vi "倒计时器.vi"() -> ()   [LabVIEW 2017]
panel:
  out "倒计时":string
  in  "停止":bool
  out "?":bool
  in  "开始倒计时":bool
  in  "定时时间选择":enum16{"20秒", "10秒", "6秒"}(ring)
  # "倒计时器"
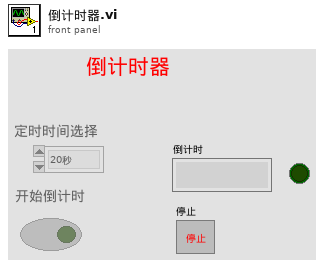
[diagram p1: front panel]
types:
  T1 = enum8{"Enabled", "Disabled", "Disabled and Grayed Out"}
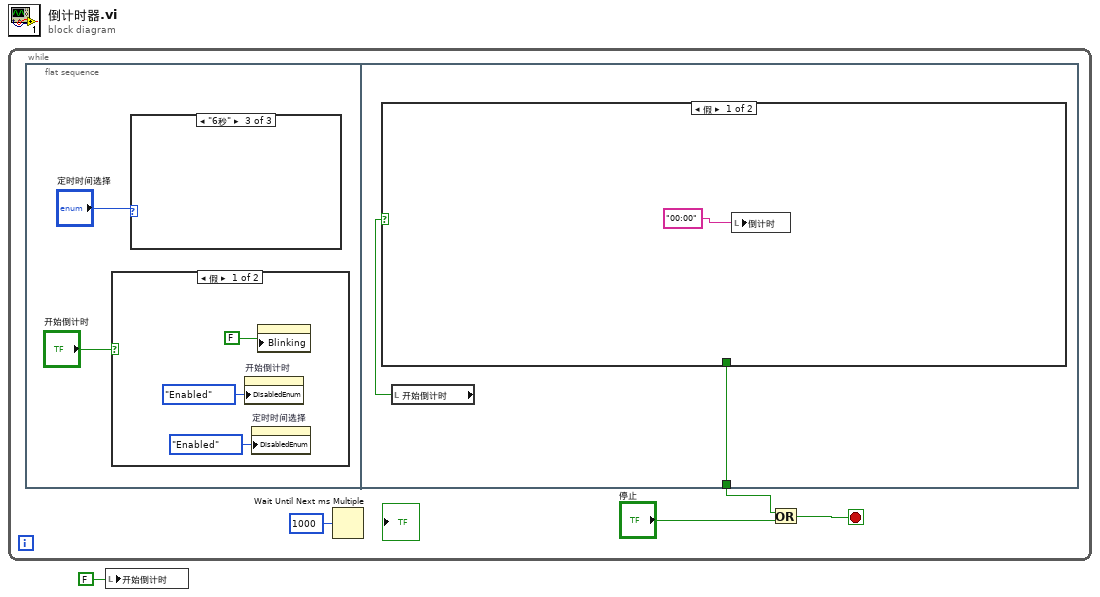
[diagram p0: block diagram]
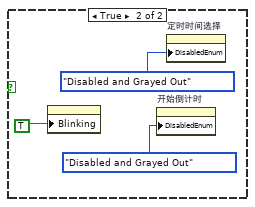
[diagram p2: hidden frame]
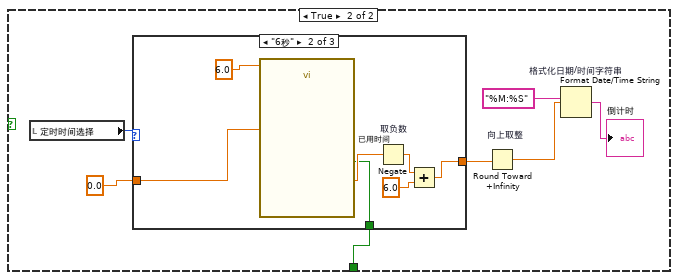
[diagram p5: hidden frame]
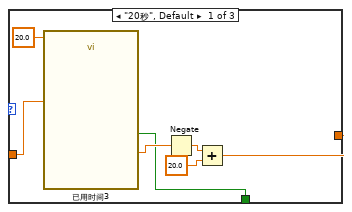
[diagram p6: hidden frame]
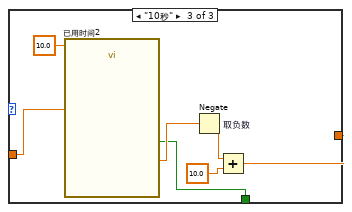
[diagram p7: hidden frame]
diagram:
  n1 = while {
    stop <- w2 stop-if-true
    n2 = flat-sequence {
      tunnel: [w14] -> w3
      frame #0 {
        n3 = case shown="假" "开始倒计时" {
          frame False {
            n4 = property on="开始倒计时" class="Bool (严格)"("DisabledEnum"=T1."Enabled" ("禁用")) -> ()  [unwired: 2 in, 2 out]
            n5 = property on="定时时间选择" class="Enum (严格)"("DisabledEnum"=T1."Enabled" ("禁用")) -> ()  [unwired: 2 in, 2 out]
            n6 = property class="Bool (严格)"("Blinking"=FALSE ("闪烁")) -> ()  [unwired: 2 in, 2 out]
          }
          frame True {
            n7 = property class="Bool (严格)"("Blinking"=TRUE ("闪烁")) -> ()  [unwired: 2 in, 2 out]
            n8 = property on="开始倒计时" class="Bool (严格)"("DisabledEnum"=T1."Disabled and Grayed Out" ("禁用")) -> ()  [unwired: 2 in, 2 out]
            n9 = property on="定时时间选择" class="Enum (严格)"("DisabledEnum"=T1."Disabled and Grayed Out" ("禁用")) -> ()  [unwired: 2 in, 2 out]
          }
        }
        n10 = case shown="\"6秒\"" "定时时间选择" {
          frame "20秒", Default {
          }
          frame "10秒" {
          }
          frame "6秒" {
          }
        }
      }
      frame #1 {
        n11 = local read "开始倒计时"() -> (w15:bool)
        n12 = case shown="假" w15 {
          tunnel: [_ w17] -> w14
          frame False {
            n13 = local write "倒计时"("00:00" ("倒计时")) -> ()
          }
          frame True {
            n14 = local read "定时时间选择"() -> (w22:enum16{"20秒", "10秒", "6秒"})
            n15 = case shown="\"6秒\"" w22 {
              tunnel: 0.0 ("Set Start Time (s)") -> [w24 w33 w38]
              tunnel: [w26 w32 w40] -> w19
              tunnel: [w25 w31 w39] -> w17
              frame "20秒", Default {
                n16 = call "已用时间3"("Time Target (s)"=20.0, "Set Start Time (s)"=w24) -> ("Elapsed Time (s)"=w29:dbl, "Time has Elapsed"=w25:bool)  [unwired: 10 in, 6 out]
                n17 = Negate(x=w29) -> (-x=w30:dbl)
                n18 = Add(x=w30, y=20.0) -> (x+y=w26:dbl)
              }
              frame "6秒" {
                n19 = call "已用时间"("Time Target (s)"=6.0, "Set Start Time (s)"=w33) -> ("Elapsed Time (s)"=w36:dbl, "Time has Elapsed"=w31:bool)  [unwired: 10 in, 6 out]
                n20 = Negate "取负数"(x=w36) -> (-x=w37:dbl)
                n21 = Add(x=w37, y=6.0) -> (x+y=w32:dbl)
              }
              frame "10秒" {
                n22 = call "已用时间2"("Time Target (s)"=10.0, "Set Start Time (s)"=w38) -> ("Elapsed Time (s)"=w43:dbl, "Time has Elapsed"=w39:bool)  [unwired: 10 in, 6 out]
                n23 = Negate "取负数"(x=w43) -> (-x=w44:dbl)
                n24 = Add(x=w44, y=10.0) -> (x+y=w40:dbl)
              }
            }
            n25 = Round Toward +Infinity "向上取整"(x=w19) -> (ceil(x): smallest int >= x=w18:dbl)
            n26 = Format Date/Time String "格式化日期/时间字符串"(time format string (%c)="%M:%S", seconds (now)=w18) -> (date/time string=→"倒计时":string)  [unwired: 1 in]
          }
        }
      }
    }
    n27 = Wait Until Next ms Multiple(millisecond multiple=u32 1000 ("毫秒倍数")) -> ()  [unwired: 1 out]
    n28 = Or(x=w3, y="停止") -> (x .or. y?=w2:bool)
  }
  n29 = local write "开始倒计时"(FALSE ("开始倒计时")) -> ()
